vi "czujnik_odbiciowy.vi"() -> ()   [LabVIEW 2014]
uses:
  <vilib>/MakerHub/LINX/Public/Peripherals/Digital/Digital Read 1 Chan.vi
  <vilib>/MakerHub/LINX/Public/Peripherals/Digital/Digital Read N Chans.vi
  <vilib>/MakerHub/LINX/Private/Local IO/LinxDigitalRead.vi
  <vilib>/MakerHub/LINX/Public/Utilities/Check Channel.vi
  <vilib>/MakerHub/LINX/Public/Utilities/Open Local.vi
  <vilib>/MakerHub/LINX/Private/Utilties/Generate Error.vi
  <vilib>/MakerHub/LINX/LMH-LINX.lvlib
panel:
  out "Liczba zmian stanu":i32
  out "Czujnik":bool
  in  "stop":bool
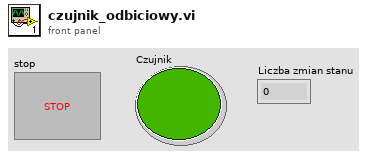
[diagram p1: front panel]
types:
  T1 = typedef "LMH-LINX.lvlib/LINX Ref.ctl" = cluster{"IO":T2, "Interface":T3, "LINX Device Config":T4}
  T2 = typedef "LMH-LINX.lvlib/Platform.ctl" = enum16{"Remote", "Local"}
  T3 = typedef "LMH-LINX.lvlib/Interface.ctl" = enum16{"Serial", "TCP"}
  T4 = typedef "LMH-LINX.lvlib/Device.lvlib/LINX Device Config.ctl" = cluster{"Interface":T3, "COM Port":refnum<visa-resource-name>, "TCP Configuration":T5, "Device Family":u8, "Device ID":u8, "Device Name":string, "TCP Ref":refnum<k5>, "Channels":T6}
  T5 = typedef "LMH-LINX.lvlib/Device.lvlib/TCP Config.ctl" = cluster{"IP Address":string, "Port":u16}
  T6 = typedef "LMH-LINX.lvlib/Channels.ctl" = cluster{"DI":u8[], "DO":u8[], "AI":u8[], "AO":u8[], "PWM":u8[], "QE":u8[], "UART":u8[], "I2C 2":u8[], "SPI":u8[], "CAN":u8[], "Servo":u8[], "AI Ref (V)":dbl, "AI Resolution (Bits)":u8, "AO Ref (V)":dbl, "AO Resolution (Bits)":u8}
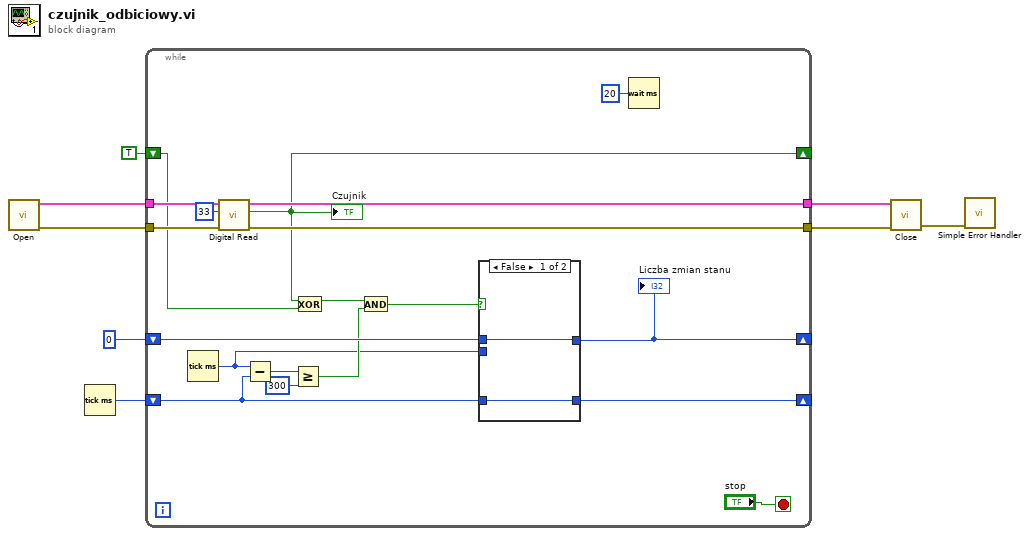
[diagram p0: block diagram]
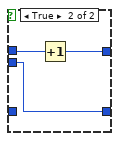
[diagram p2: hidden frame]
diagram:
  n1 = call-poly <vilib>:"Open.vi"() -> ("Error Out"=w6:errorcluster, "LINX Resource"=w8:T1)  [unwired: 9 in, 1 out]
  n2 = Tick Count (ms)() -> (millisecond timer value=w1:u32)
  n3 = while {
    tunnel: w8 -> [w25]
    tunnel: [w24] -> w7
    tunnel: w6 -> [w23]
    tunnel: [w22] -> w5
    shift-right: [w19] -> _
    shift-left: TRUE ("DI Value") -> [w20]
    shift-right: [w17] -> _
    shift-left: 0 -> [w18]
    shift-right: [w9] -> _
    shift-left: w1 -> [w11]
    stop <- "stop" stop-if-true
    n4 = Tick Count (ms)() -> (millisecond timer value=w10:u32)
    n5 = call-poly <vilib>:"Digital Read.vi"("Error In"=w23, "DI Channel"=u8 33, "LINX Resource"=w25) -> ("Error Out"=w22:errorcluster, "DI Value"=w19:bool, "LINX Resource"=w24:T1)  [unwired: 6 in]
    "Czujnik" <- w19
    n6 = Subtract(x=w10, y=w11) -> (x-y=w16:u32)
    n7 = Greater Or Equal?(x=w16, y=u32 300) -> (x >= y?=w13:bool)
    n8 = Exclusive Or(1:w20, 2:w19) -> (0:w14:bool)
    n9 = And(x=w14, y=w13) -> (x .and. y?=w12:bool)
    n10 = case shown="False" w12 {
      tunnel: w18 -> [w29 w32]
      tunnel: [w29 w31] -> w17
      tunnel: w11 -> [w28 _]
      tunnel: w10 -> [_ w30]
      tunnel: [w28 w30] -> w9
      frame False {
      }
      frame True {
        n11 = Increment(x=w32) -> (x+1=w31:i32)
      }
    }
    "Liczba zmian stanu" <- w17
    n12 = Wait (ms)(milliseconds to wait=u32 20) -> ()  [unwired: 1 out]
  }
  n13 = call <vilib>:"Close.vi"("Error In"=w5, "LINX Resource"=w7) -> ("Error Out"=w4:errorcluster)  [unwired: 9 in]
  n14 = call <vilib>:"Simple Error Handler.vi"("error in (no error)"=w4) -> ()  [unwired: 4 in, 5 out]
